vi "example-just-read.vi"() -> ()   [LabVIEW 2024]
uses:
  cfitsio-bitpix.ctl
  cfitsio-datatypes.ctl
  gfitsio.lvlib
panel:
  out "Final Error":errorcluster
  out "data":dbl[][][](array[numeric])
  out "Array":dbl[][][](array[numeric])
  out "error out 3":errorcluster
  out "error out 2":errorcluster
  out "cfitsio datatype":T1 items=["TBIT"=1, "TBYTE  (U8)"=11, "TSBYTE  (I8)"=12, "TLOGICAL"=14, "TSTRING"=16, "TUSHORT  (U16)"=20, "TSHORT  (I16)"=21, "TUINT"=31, "TULONG  (U32)"=40, "TLONG  (I32)"=41, "TFLOAT  (SGL)"=42, "TLONGLONG  (I64)"=81, "TDOUBLE  (DBL)"=82, "TCOMPLEX  (CSG)"=83, "TDOUBLECOMPLEX  (CDB)"=163]
  out "bitpix":T2 items=["<invalid type>"=0, "BYTE_IMG  (U8)"=8, "SHORT_IMG  (I16)"=16, "USHORT_IMG  (U16)"=20, "LONG_IMG  (I32)"=32, "ULONG_IMG  (U32)"=40, "FLOAT_IMG  (SGL)"=-32, "DOUBLE_IMG  (DBL)"=-64]
  out "error out":errorcluster
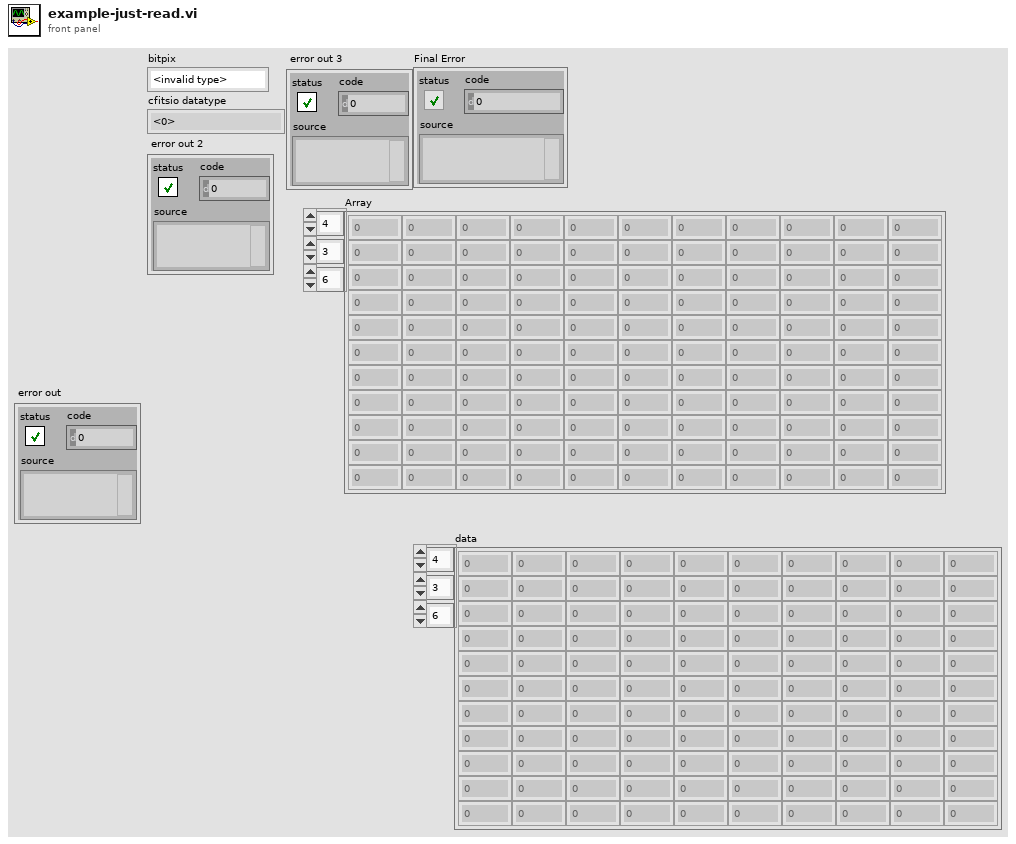
[diagram p1: front panel]
types:
  T1 = typedef "gfitsio.lvlib/cfitsio-datatypes.ctl" = i32
  T2 = typedef "gfitsio.lvlib/cfitsio-bitpix.ctl" = i32
  T3 = enum16{"open", "open or create", "create or replace", "create", "open (read only)"}
  T4 = typedef "gfitsio.lvlib/gfitsio-refnum.ctl" = refnum<k1>
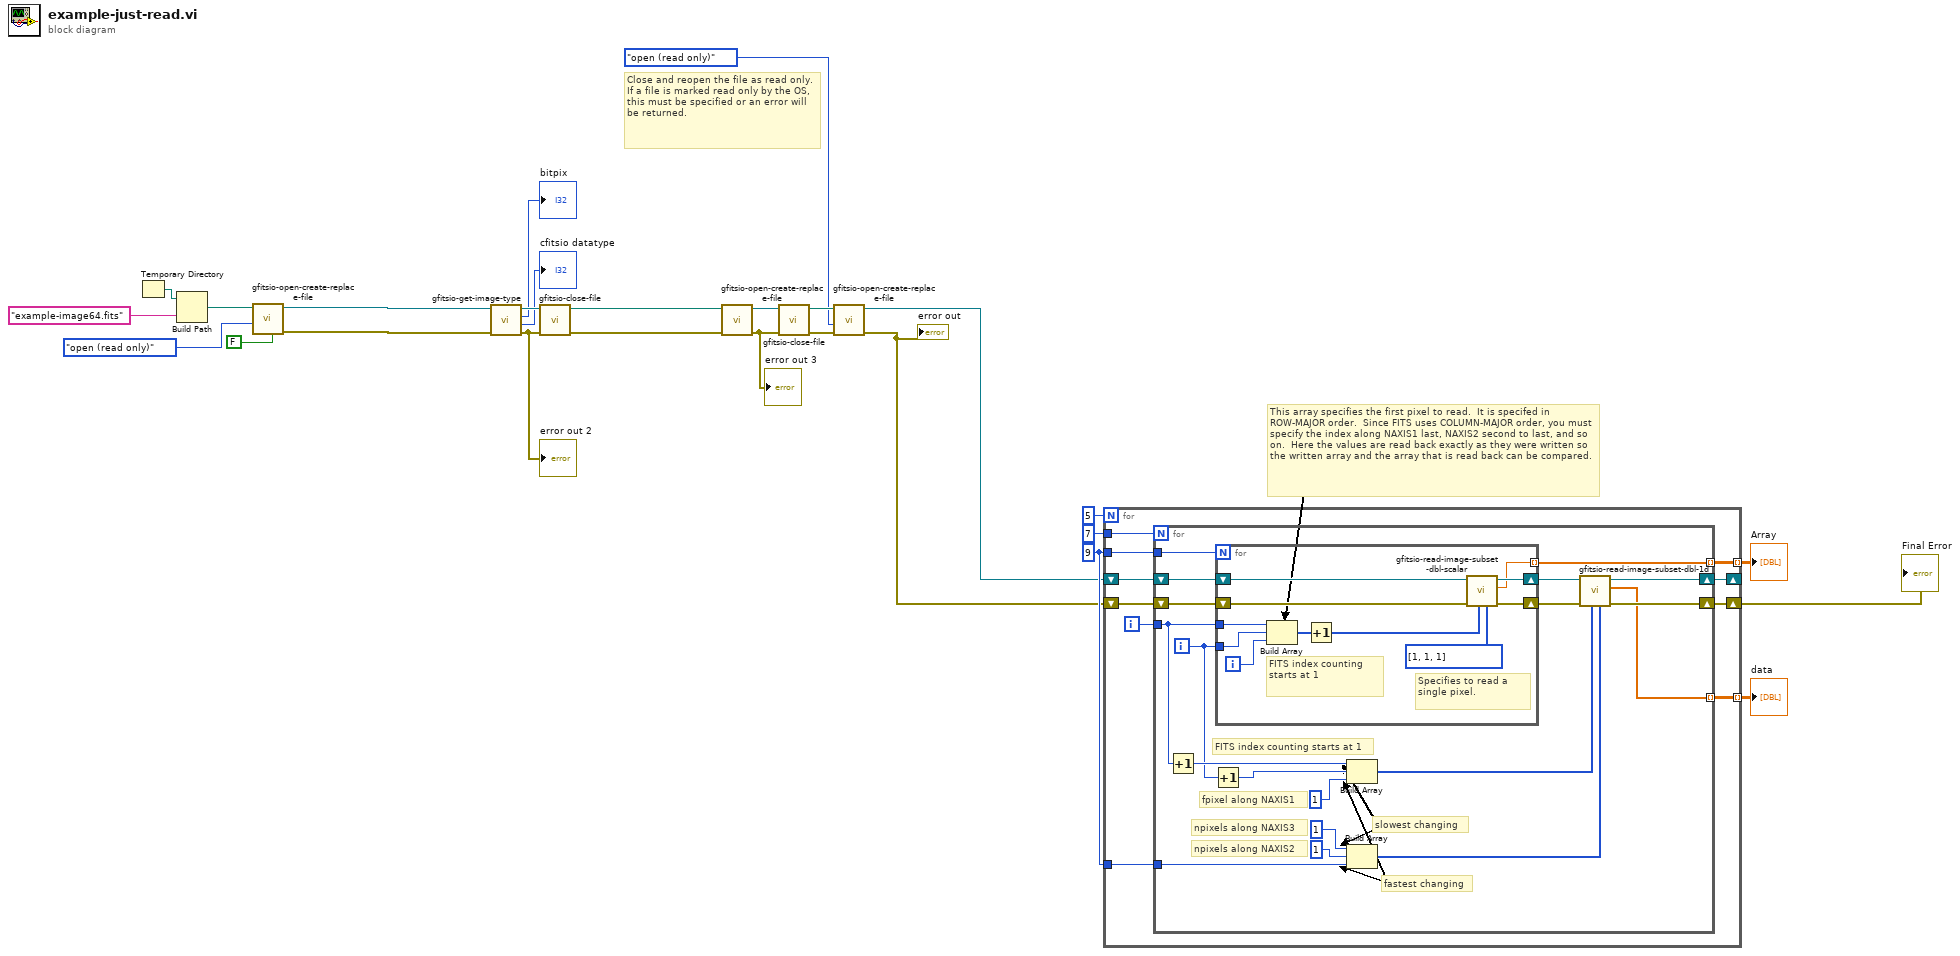
[diagram p0: block diagram]
diagram:
  w6 = 9
  # "This array specifies the first pixel to read.  It is specifed in ROW-MAJOR order.  Since FITS uses COLUMN-MAJOR order, you must specify the index along NAXIS1 last, NAXIS2 second to last, and so on.  Here the values are read back exactly as they were written so the written array and the array that is read back can be compared."
  # "Close and reopen the file as read only.  If a file is marked read only by the OS, this must be specified or an error will be returned."
  n1 = Temporary Directory() -> (w22:path)
  n2 = Build Path(base path=w22, name or relative path="example-image64.fits") -> (appended path=w20:path)
  n3 = call "gfitsio-open-create-replace-file.vi"("advisory dialog? (display:T)"=FALSE, "function (open)"=T3."open (read only)", "file path (dialog if empty)"=w20) -> ("error out"=w14:errorcluster, "gfits refnum"=w12:T4)  [unwired: 6 in, 1 out]
  n4 = call "gfitsio-get-image-type.vi"("error in (no error)"=w14, "gfits refnum"=w12) -> ("error out"=w13:errorcluster, "cfitsio datatype"=→"cfitsio datatype":T1, "bitpix"=→"bitpix":T2, "dup gfits refnum"=w11:T4)  [unwired: 6 in]
  "error out 2" <- w13
  n5 = call "gfitsio-close-file.vi"("error in (no error)"=w13, "gfits refnum"=w11) -> ("error out"=w24:errorcluster, "Path"=w23:path)  [unwired: 8 in]
  n6 = call "gfitsio-open-create-replace-file.vi"("error in (no error)"=w24, "file path (dialog if empty)"=w23) -> ("error out"=w16:errorcluster, "gfits refnum"=w17:T4)  [unwired: 7 in, 1 out]
  "error out 3" <- w16
  n7 = call "gfitsio-close-file.vi"("error in (no error)"=w16, "gfits refnum"=w17) -> ("error out"=w18:errorcluster, "Path"=w19:path)  [unwired: 8 in]
  n8 = call "gfitsio-open-create-replace-file.vi"("error in (no error)"=w18, "function (open)"=T3."open (read only)", "file path (dialog if empty)"=w19) -> ("error out"=w4:errorcluster, "gfits refnum"=w5:T4)  [unwired: 6 in, 1 out]
  "error out" <- w4
  n9 = for {
    N: 5 -> [_]
    shift-right: [w35] -> w1
    shift-left: w4 -> [w36]
    shift-right: [w33] -> _
    shift-left: w5 -> [w34]
    tunnel: w6 -> [w32]
    tunnel: 7 -> [w31]
    tunnel: [w29] -> w3 mode=indexing
    tunnel: w6 -> [w28]
    tunnel: [w27] -> w2 mode=indexing
    i -> [w30]
    n10 = for {
      N: w31 -> [_]
      shift-right: [w48] -> w35
      shift-left: w36 -> [w55]
      shift-right: [w49] -> w33
      shift-left: w34 -> [w54]
      tunnel: w32 -> [w53]
      tunnel: w30 -> [w40]
      tunnel: [w52] -> w29 mode=indexing
      tunnel: w28 -> [w47]
      tunnel: [w43] -> w27 mode=indexing
      i -> [w38]
      # "fastest changing"
      # "slowest changing"
      # "fpixel along NAXIS1"
      # "npixels along NAXIS2"
      # "npixels along NAXIS3"
      # "FITS index counting starts at 1"
      n11 = Increment(x=w40) -> (x+1=w39:i32)
      n12 = Increment(x=w38) -> (x+1=w37:i32)
      n13 = for {
        N: w53 -> [_]
        shift-right: [w65] -> w51
        shift-left: w55 -> [w66]
        shift-right: [w63] -> w50
        shift-left: w54 -> [w64]
        tunnel: w38 -> [w58]
        tunnel: w40 -> [w57]
        tunnel: [w56] -> w52 mode=indexing
        i -> [w59]
        # "Specifies to read a single pixel."
        # "FITS index counting starts at 1"
        n14 = Build Array(w57, w58, w59) -> (w61:i32[])
        n15 = Increment(x=w61) -> (x+1=w60:i32[])
        n16 = call "gfitsio-read-image-subset-dbl-scalar.vi"("npixels (rest)"=i32[] [1, 1, 1], "fpixel (origin)"=w60, "error in (no error)"=w66, "gfits refnum"=w64) -> ("error out"=w65:errorcluster, "data"=w56:dbl, "dup gfits refnum"=w63:T4)  [unwired: 5 in]
      }
      n17 = Build Array(w39, w37, 1 ("element")) -> (w41:i32[])
      n18 = Build Array(1 ("element"), 1 ("element"), w47) -> (w42:i32[])
      n19 = call "gfitsio-read-image-subset-dbl-1d.vi"("npixels (rest)"=w42, "fpixel (origin)"=w41, "error in (no error)"=w51, "gfits refnum"=w50) -> ("error out"=w48:errorcluster, "data"=w43:dbl[], "dup gfits refnum"=w49:T4)  [unwired: 5 in]
    }
  }
  "Array" <- w3
  "data" <- w2
  "Final Error" <- w1
